vi "new.vi"() -> ()   [LabVIEW 2011]
panel:
  in  "停止":bool
  out "数值 3":dbl
  in  "数值 2":dbl
  in  "数值":dbl
  # "这是一个测试加法的子面板"
  # "+"
  # "="
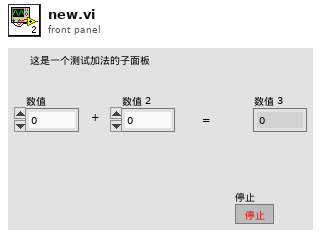
[diagram p1: front panel]
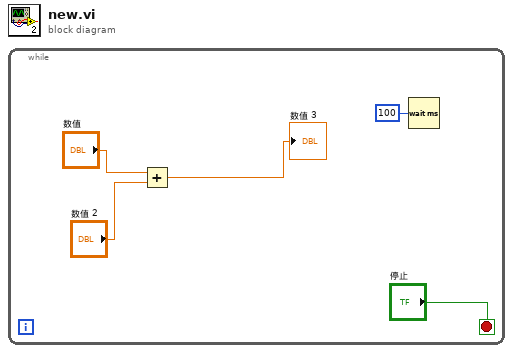
[diagram p0: block diagram]
diagram:
  n1 = while {
    stop <- "停止" stop-if-true
    n2 = Add(x="数值", y="数值 2") -> (x+y=→"数值 3":dbl)
    n3 = Wait (ms)(milliseconds to wait=u32 100 ("等待时间（毫秒）")) -> ()  [unwired: 1 out]
  }
